vi "PWM_SetValue.vi"(5 "PWM":T1=1 items=["Invalid"=0, "PWM1"=1, "PWM2"=2, "PWM9"=9, "PWM10"=10], 7 "High (uSec)":u32, 9 "Period (uSec)":u32, 11 "error in":errorcluster) -> (15 "error out":errorcluster)   [LabVIEW 2009, in "PWM.lvlib"]
uses:
  PWM.lvlib
  <vilib>/rvi/interface/nirviReadWriteControl/nirviReadWriteControl.xnode
  RobotFPGA.vi
  FPGA Bitfiles/scmproject.lvproj_FPGA Target_RobotFPGA.vi.lvbitx
  <vilib>/LabVIEW Targets/FPGA/Rio/nirio_HostInterface/nirio_WriteBig.vi
  <vilib>/rvi/errors/niLvFpgaWhatHappensToTopLevelVI.ctl
  <vilib>/rvi/interface/common/niFpgaNodeNameForErrorReporting.ctl
  <vilib>/rvi/errors/niLvFpgaAdjustHostInterfaceError.vi
  FPGA.lvlib
  PWM_Name.ctl
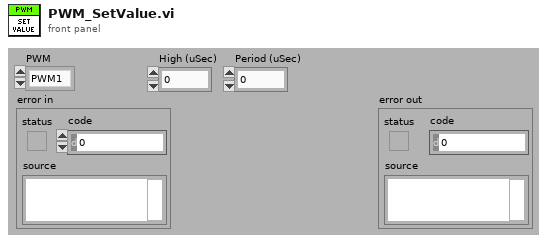
[diagram p1: front panel]
types:
  T1 = typedef "PWM.lvlib/PWM_Name.ctl" = u16
  T2 = typedef "niFpgaNodeNameForErrorReporting.ctl" = enum16{"Open FPGA VI Reference", "Read/Write Control", "Invoke Method: Abort", "Invoke Method: Acknowledge IRQ", "Invoke Method: Download", "Invoke Method: FIFO.Configure", "Invoke Method: FIFO.Read", "Invoke Method: FIFO.Start", "Invoke Method: FIFO.Stop", "Invoke Method: FIFO.Write", "Invoke Method: Reset", "Invoke Method: Run", "Invoke Method: Wait on IRQ", "Close FPGA VI Reference"}
  T3 = typedef "niLvFpgaWhatHappensToTopLevelVI.ctl" = enum16{"top level VI scripted behind XNode", "top level VI inlined behind XNode"}
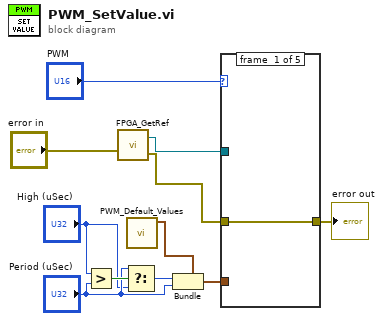
[diagram p0: block diagram]
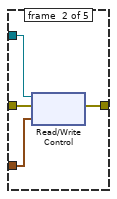
[diagram p2: hidden frame]
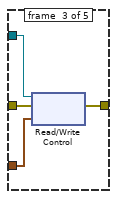
[diagram p3: hidden frame]
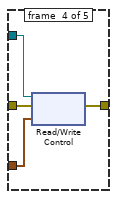
[diagram p4: hidden frame]
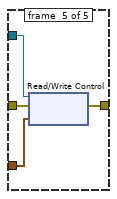
[diagram p5: hidden frame]
diagram:
  n1 = Greater?(x="High (uSec)", y="Period (uSec)") -> (0:w7:bool)
  n2 = call "FPGA_GetRef.vi"("error in (no error)"="error in") -> ("error out"=w1:errorcluster, "FPGA_Ref"=w3:refnum<k20>)  [unwired: 1 in]
  n3 = Select(t="Period (uSec)", s=w7, f="High (uSec)") -> (s? t:f=w8:u32)
  n4 = call "PWM_Default_Values.vi"() -> ("PWM_default"=w9:cluster{"High (uSec)":u32, "Period (uSec)":u32})  [unwired: 11 in]
  n5 = Bundle(cluster=w9, "High (uSec)"=w8, "Period (uSec)"="Period (uSec)") -> (w10:cluster{"High (uSec)":u32, "Period (uSec)":u32})
  n6 = case shown="1" "PWM" {
    tunnel: w3 -> [w13 w14 w46 w78 w110]
    tunnel: w1 -> [w12 w17 w49 w81 w113]
    tunnel: [w12 w16 w48 w80 w112] -> w4
    tunnel: w10 -> [_ w15 w47 w79 w111]
    frame #0 {
    }
    frame #1 {
      n7 = xnode "Read/Write Control"("FPGA VI Reference In"=w14, "error in"=w17, "PWM1"=w15) -> ("error out"=w16:errorcluster)  [unwired: 1 out]
    }
    frame #2 {
      n8 = xnode "Read/Write Control"("FPGA VI Reference In"=w46, "error in"=w49, "PWM2"=w47) -> ("FPGA VI Reference Out"=w45:refnum<k20>, "error out"=w48:errorcluster)
    }
    frame #3 {
      n9 = xnode "Read/Write Control"("FPGA VI Reference In"=w78, "error in"=w81, "PWM9"=w79) -> ("FPGA VI Reference Out"=w77:refnum<k20>, "error out"=w80:errorcluster)
    }
    frame #4 {
      n10 = xnode "Read/Write Control"("FPGA VI Reference In"=w110, "error in"=w113, "PWM10"=w111) -> ("FPGA VI Reference Out"=w109:refnum<k20>, "error out"=w112:errorcluster)
    }
  }
  "error out" <- w4
